vi "CmdConsole.Stand Alone Run and Wait with Timeout.vi"(8 "error in (no error)":errorcluster, 9 "Timeout(s)":dbl=1.0, 10 "Args":string, 11 "Exe":path) -> (0 "error out":errorcluster, 1 "Std Error":string, 2 "Std Out":string, 4 "RtnCode":i32, 5 "Duration":dbl)   [LabVIEW 2018, in "CmdConsole.lvclass"]
uses:
  CmdConsole.lvclass
  CmdConsole.lvclass/CmdConsole.ctl
  Errors/Error.Error Code List.ctl
  <vilib>/KATE/Time/Time Utils.lvlib
panel:
  out "HasExited":bool
  out "WaitForExit":bool
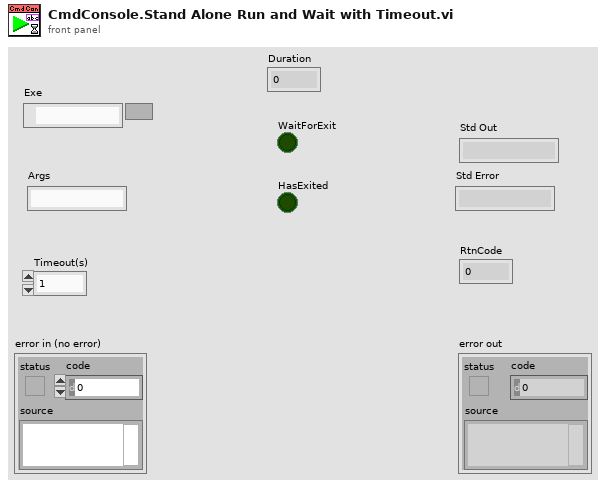
[diagram p1: front panel]
types:
  T1 = cluster{"StdOut":string, "StdErr":string, "RtnCode":i32}
  T2 = typedef "Error.Error Code List.ctl" = i32
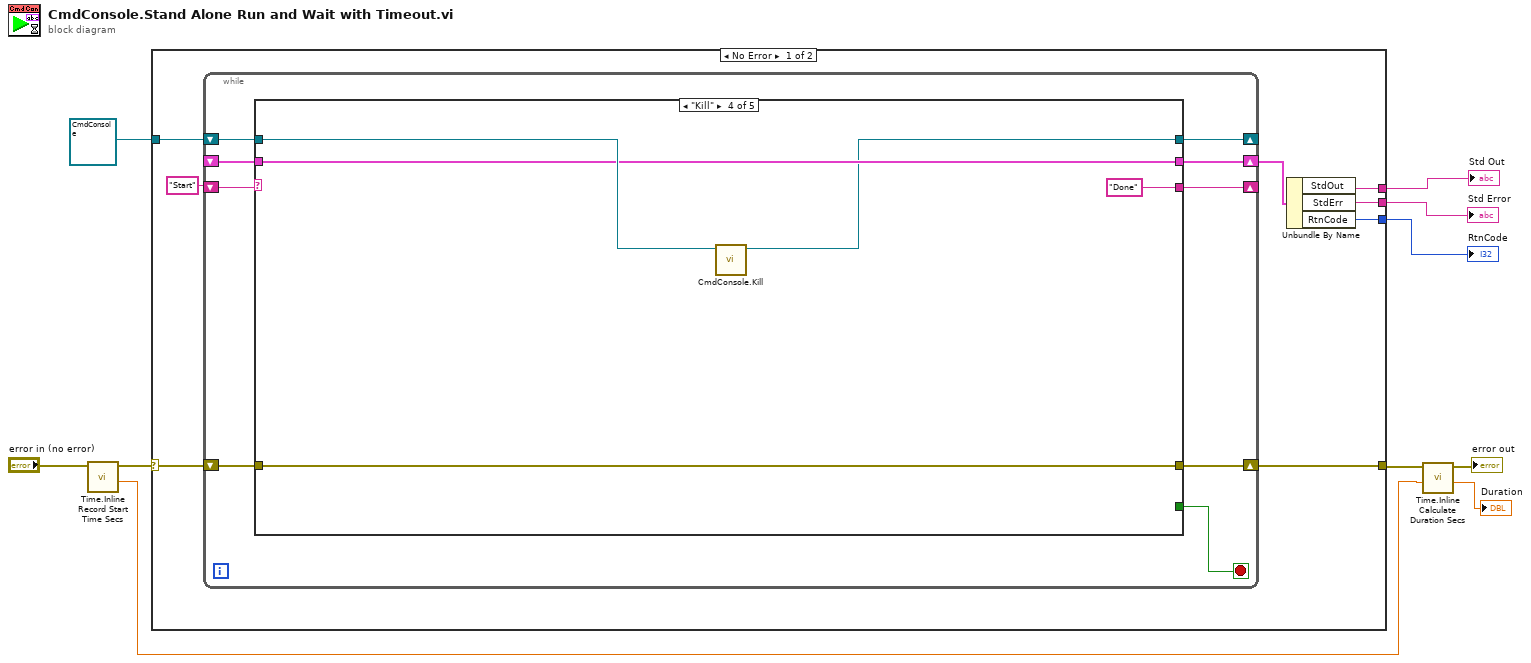
[diagram p0: block diagram]
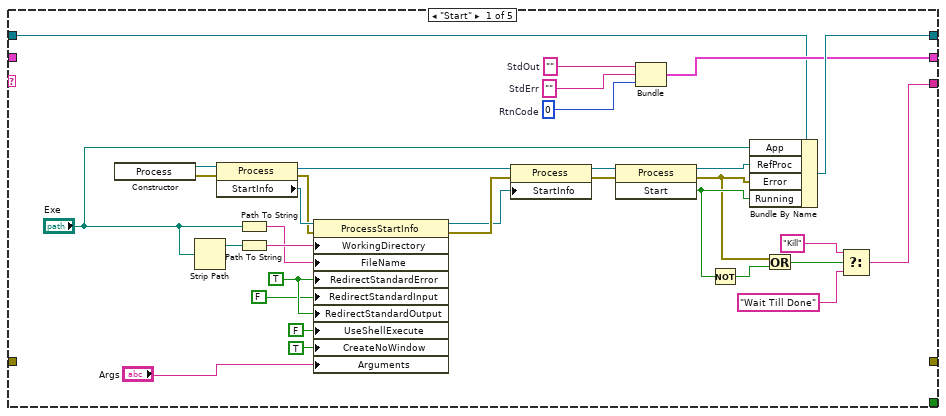
[diagram p2: hidden frame]
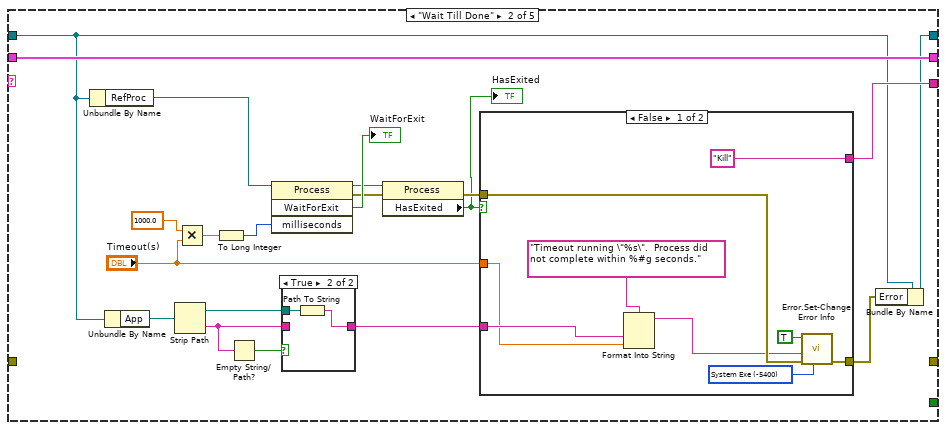
[diagram p3: hidden frame]
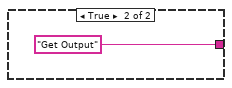
[diagram p5: hidden frame]
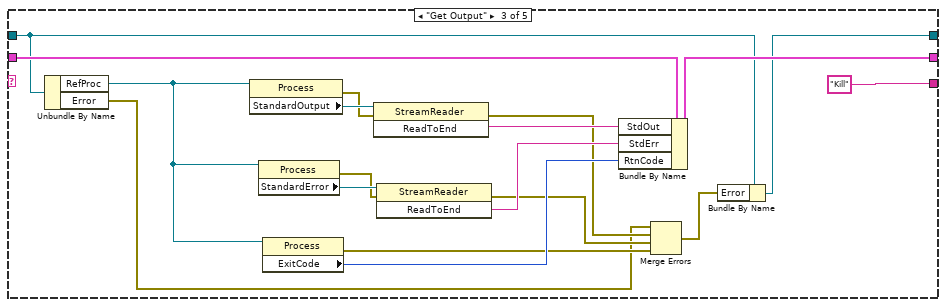
[diagram p6: hidden frame]
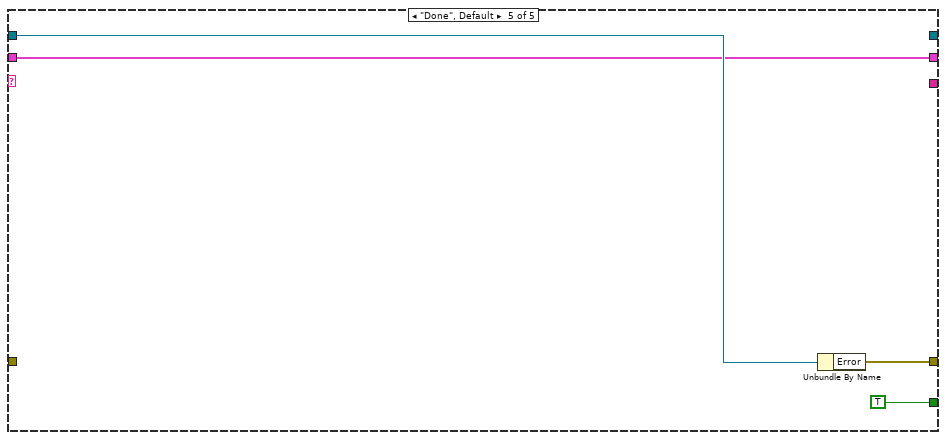
[diagram p7: hidden frame]
diagram:
  n1 = call <vilib>:"Time.Inline Record Start Time Secs.vi"("Error In Upper"="error in (no error)") -> ("Start(s)"=w2:dbl, "Error Out Upper"=w5:errorcluster)  [unwired: 8 in, 1 out]
  n2 = case shown="No Error" w5 {
    selector: w5 -> [w15 w120]
    tunnel: [w16 w120] -> w3
    tunnel: refnum<class "CmdConsole.lvclass"> refnum ("CmdConsole in") -> [w18 _]
    tunnel: [w14 _] -> w9
    tunnel: [w12 _] -> w8
    tunnel: [w11 _] -> w7
    frame No Error {
      n3 = while {
        shift-right: [w26] -> _
        shift-left: w18 -> [w27]
        shift-right: [w24] -> _
        shift-left: "Start" -> [w25]
        shift-right: [w22] -> w16
        shift-left: w15 -> [w19]
        shift-right: [w21] -> w13
        shift-left: _ -> [w20]
        stop <- w23 stop-if-true
        n4 = case shown="\"Kill\"" w25 {
          tunnel: w27 -> [w30 w65 w101 w115 w118]
          tunnel: [w44 w64 w100 w111 _] -> w26
          tunnel: [w36 w75 "Kill" "Done" _] -> w24
          tunnel: [_ _ _ _ TRUE] -> w23
          tunnel: [_ _ _ w112 w117] -> w22
          tunnel: [w31 w71 w106 w113 w116] -> w21
          tunnel: w20 -> [_ w71 w107 w113 w116]
          tunnel: w19 -> [_ _ _ w112 _]
          frame "Start" {
            w32 = 0  # RtnCode
            w33 = ""  # StdErr
            w34 = ""  # StdOut
            w45 = TRUE ("UseShellExecute")
            n5 = constructor class="Process"() -> (reference out=w59:refnum<k24>, error out=w58:errorcluster)  [unwired: 3 in, 1 out]
            n6 = Strip Path(path="Exe") -> (stripped path=w48:path)  [unwired: 1 out]
            n7 = property class="Process"(reference=w59, error in=w58) -> (reference out=w51:refnum<k24>, error out=w52:errorcluster, "StartInfo"=w57:refnum<k24>)
            n8 = Path To String(path="Exe") -> (string=w46:string)
            n9 = Path To String(path=w48) -> (string=w47:string)
            n10 = property class="ProcessStartInfo"(reference=w57, error in=w52, "WorkingDirectory"=w47, "FileName"=w46, "RedirectStandardError"=w45, "RedirectStandardInput"=FALSE ("UseShellExecute"), "RedirectStandardOutput"=w45, "UseShellExecute"=FALSE, "CreateNoWindow"=TRUE, "Arguments"="Args") -> (reference out=w53:refnum<k24>, error out=w54:errorcluster)
            n11 = property class="Process"(reference=w51, error in=w54, "StartInfo"=w53) -> (reference out=w50:refnum<k24>, error out=w49:errorcluster)
            n12 = invoke class="Process" method="Start"(reference=w50, error in=w49) -> (reference out=w43:refnum<k24>, error out=w40:errorcluster, "Start"=w42:bool)  [unwired: 1 in]
            n13 = Bundle("StdOut"=w34, "StdErr"=w33, "RtnCode"=w32) -> (w31:T1)  [unwired: 1 in]
            n14 = Not(x=w42) -> (.not. x?=w41:bool)
            n15 = Bundle By Name(cluster=w30, "App"="Exe", "RefProc"=w43, "Error"=w40, "Running"=w42) -> (w44:refnum<class "CmdConsole.lvclass">)
            n16 = Or(x=w40, y=w41) -> (x .or. y?=w39:bool)
            n17 = Select(t="Kill", s=w39, f="Wait Till Done") -> (s? t:f=w36:string)
          }
          frame "Wait Till Done" {
            n18 = Unbundle By Name(w65) -> ("RefProc"=w79:refnum<k24>)
            n19 = Unbundle By Name(w65) -> ("App"=w74:path)
            n20 = Strip Path(path=w74) -> (stripped path=w62:path, name=w60:string)
            n21 = Multiply(x=1000.0 ("y"), y="Timeout(s)") -> (x*y=w78:dbl)
            n22 = To Long Integer(number=w78) -> (32bit integer=w77:i32)
            n23 = Empty String/Path?(string/path=w60) -> (empty?=w63:bool)
            n24 = invoke class="Process" method="WaitForExit"(reference=w79, "milliseconds"=w77) -> (reference out=w70:refnum<k24>, error out=w68:errorcluster, "WaitForExit"=→"WaitForExit":bool)  [unwired: 2 in, 1 out]
            n25 = case shown="True" w63 {
              tunnel: w62 -> [_ w82]
              tunnel: [w80 w81] -> w61
              tunnel: w60 -> [w80 _]
              frame False {
              }
              frame True {
                n26 = Path To String(path=w82) -> (string=w81:string)
              }
            }
            n27 = property class="Process"(reference=w70, error in=w68) -> (error out=w69:errorcluster, "HasExited"=w67:bool)  [unwired: 1 out]
            "HasExited" <- w67
            n28 = case shown="False" w67 {
              tunnel: ["Kill" "Get Output"] -> w75
              tunnel: w61 -> [w86 _]
              tunnel: w69 -> [w89 _]
              tunnel: [w88 _] -> w66
              tunnel: "Timeout(s)" -> [w85 _]
              frame False {
                w83 = T2 -5400 items=["No Error"=0, "Abort"=-2, "Misc"=-5000, "Fixture Error"=-5100, "File IO - General"=-5200, "FIle IO - Config Error"=-5201, "Instrument - General"=-5300, "Instrument - Serial Com"=-5301, "Instrument - Camera"=-5302, "Instrument - PS"=-5303, "Instrument - Oscilloscope"=-5304, "Instrument - Function Gen"=-5305, "Instrument - Load"=-5306, "Instrument - Meter"=-5307, "Instrument - Power Control"=-5308, "Instrument - Motion"=-5309, "Instrument - RF"=-5310, "System Exe"=-5400, "Image Processing"=-5500, "Communication"=-5600, "Script - Syntax Error"=-6000, "Script - Invalid Name or Param"=-6100, "Script - Timeout"=-6200, "Invalid Data"=-6300, "FW Update Error"=-6500] ("Std Code")
                n29 = Format Into String(format string="Timeout running \"%s\".  Process did not complete within %#g seconds.", w86, w85) -> (resulting string=w84:string)  [unwired: 2 in, 1 out]
                n30 = call "Error.Set-Change Error Info.vi"("Std Code"=w83, "error in"=w89, "Description"=w84, "Set Error"=TRUE) -> ("error out"=w88:errorcluster)  [unwired: 7 in]
              }
              frame True {
              }
            }
            n31 = Bundle By Name(cluster=w65, "Error"=w66) -> (w64:refnum<class "CmdConsole.lvclass">)
          }
          frame "Get Output" {
            n32 = Unbundle By Name(w101) -> ("RefProc"=w103:refnum<k24>, "Error"=w93:errorcluster)
            n33 = property class="Process"(reference=w103) -> (error out=w99:errorcluster, "StandardOutput"=w109:refnum<k24>)  [unwired: 1 in, 1 out]
            n34 = property class="Process"(reference=w103) -> (error out=w98:errorcluster, "StandardError"=w105:refnum<k24>)  [unwired: 1 in, 1 out]
            n35 = property class="Process"(reference=w103) -> (error out=w97:errorcluster, "ExitCode"=w102:i32)  [unwired: 1 in, 1 out]
            n36 = invoke class="StreamReader" method="ReadToEnd"(reference=w109, error in=w99) -> (error out=w95:errorcluster, "ReadToEnd"=w108:string)  [unwired: 1 in, 1 out]
            n37 = invoke class="StreamReader" method="ReadToEnd"(reference=w105, error in=w98) -> (error out=w96:errorcluster, "ReadToEnd"=w104:string)  [unwired: 1 in, 1 out]
            n38 = Bundle By Name(cluster=w107, "StdOut"=w108, "StdErr"=w104, "RtnCode"=w102) -> (w106:T1)
            n39 = Merge Errors(w93, w95, w96, w97) -> (w94:errorcluster)
            n40 = Bundle By Name(cluster=w101, "Error"=w94) -> (w100:refnum<class "CmdConsole.lvclass">)
          }
          frame "Kill" {
            n41 = call "CmdConsole.Kill.vi"("CmdConsole in"=w115) -> ("CmdConsole out"=w111:refnum<class "CmdConsole.lvclass">)  [unwired: 9 in, 1 out]
          }
          frame "Done", Default {
            n42 = Unbundle By Name(w118) -> ("Error"=w117:errorcluster)
          }
        }
      }
      n43 = Unbundle By Name(w13) -> ("StdOut"=w14:string, "StdErr"=w12:string, "RtnCode"=w11:i32)
    }
    frame Error {
    }
  }
  "Std Error" <- w8
  "RtnCode" <- w7
  "Std Out" <- w9
  n44 = call <vilib>:"Time.Inline Calculate Duration Secs.vi"("Start(Sec)"=w2, "Error In Top"=w3) -> ("Duration(s)"=→"Duration":dbl, "Error Out Top"=→"error out":errorcluster)  [unwired: 7 in, 1 out]
